vi "module-07-sample-7-1-ALT2.vi"() -> ()   [LabVIEW 2019]
uses:
  CubeGrabeState_ENUM.ctl
  <vilib>/Rock Robotics/WPI/ThirdParty/JAS_Junk/TrajLib/Trajectory_Library.lvlib
  samples-common-library/Ctrl_Training_Library_Protected/CtrlTrainingLibary_Protected.lvlib
panel:
  in  "Tab Control":T1(tab)
  in  "Driver Gather Cube":bool
  in  "Driver Cancel Button":bool
  out "Request GO":bool
  out "Digital State Chart":cluster{dbl, dbl, dbl, dbl, dbl, dbl}(graph)
  out "Ready":bool
  out "Arm Extend Cmd":bool
  out "Hand Close Cmd":bool
  out "State":i32
  out "Done Time":dbl format="%20.3f"
  out "Cur Time":dbl format="%20.3f"
  out "State Text":T2
  # "Training Sample 7.1  ALT 2\nState Machine"
  # "F1"
  # "F2"
  # "NOTE: Outer loop not shown for simplicity"
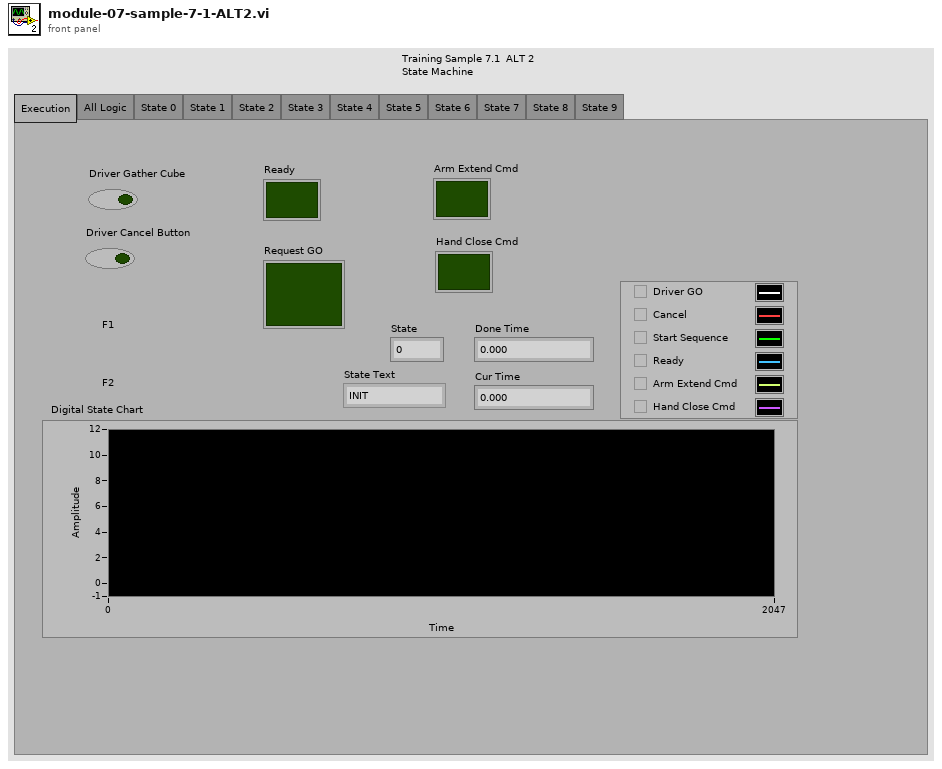
[diagram p1: front panel]
types:
  T1 = enum32{"Execution", "All Logic", "State 0", "State 1", "State 2", "State 3", "State 4", "State 5", "State 6", "State 7", "State 8", "State 9"}
  T2 = typedef "CubeGrabeState_ENUM.ctl" = enum16{"INIT", "ArmExtend", "ArmExtendWait", "HandClose", "HandCloseWait", "ArmRetract", "ArmRetractWait", "HandOpen", "HandOpenWait", "Ready"}
  T3 = typedef "Trajectory_Library.lvlib/TIMER.ctl" = cluster{"StartTime":dbl, "Accumulated TIme":dbl, "Running":bool, "semaphore":T4}
  T4 = typedef "Semaphore RefNum" = refnum<k1>
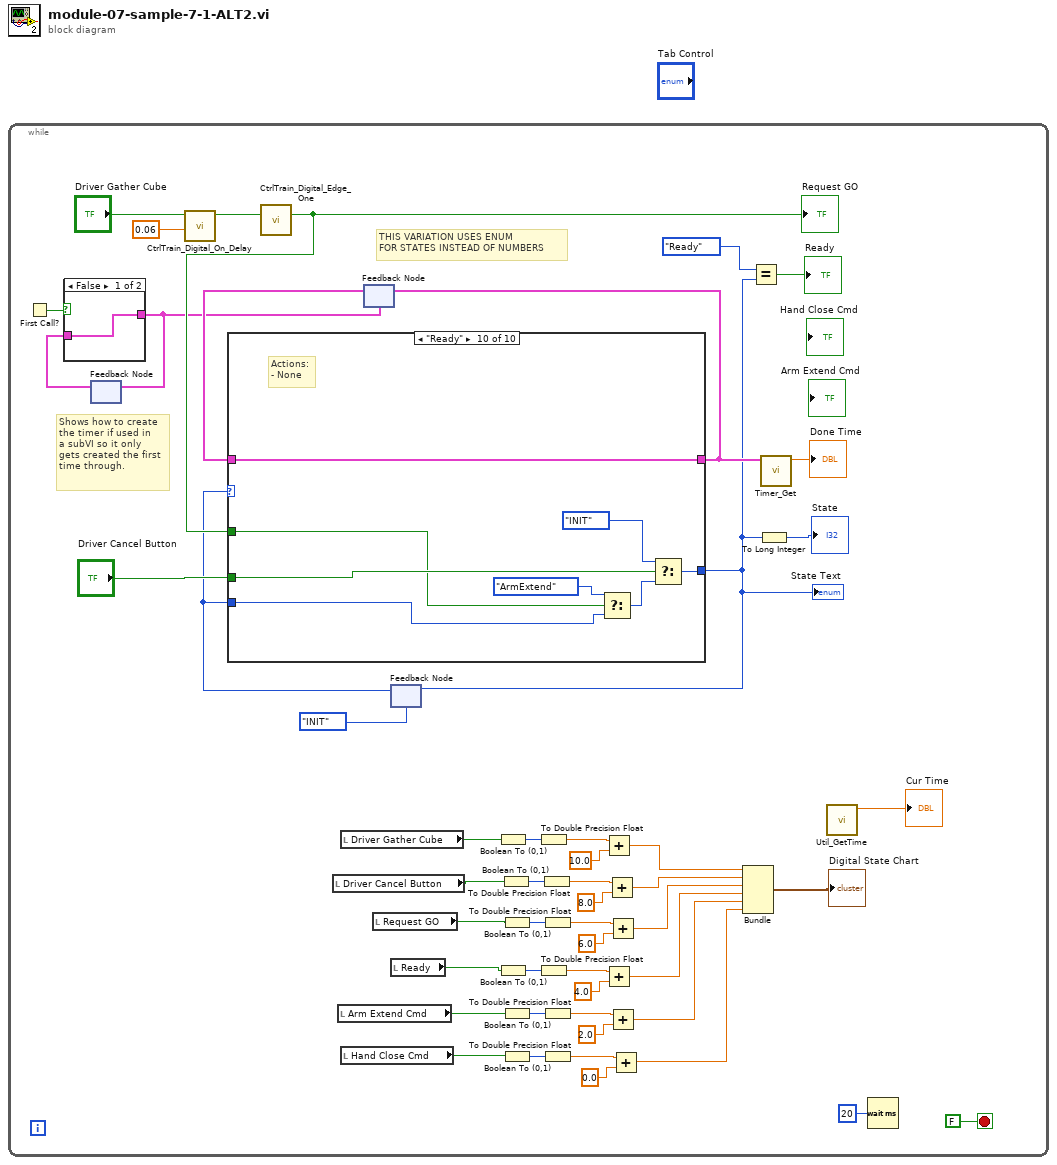
[diagram p0: block diagram]
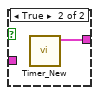
[diagram p2: hidden frame]
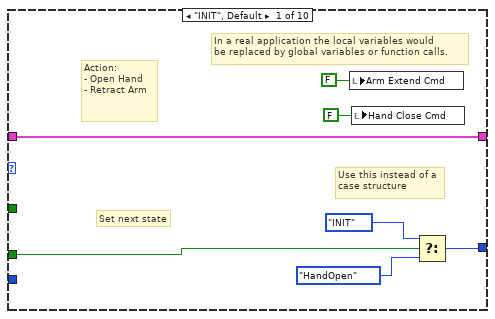
[diagram p3: hidden frame]
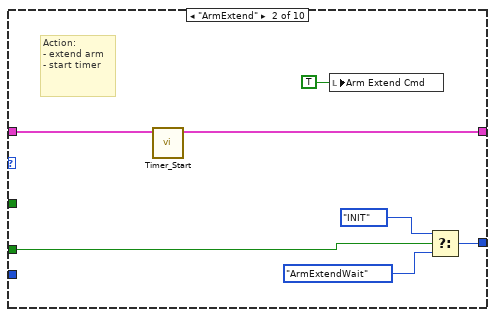
[diagram p4: hidden frame]
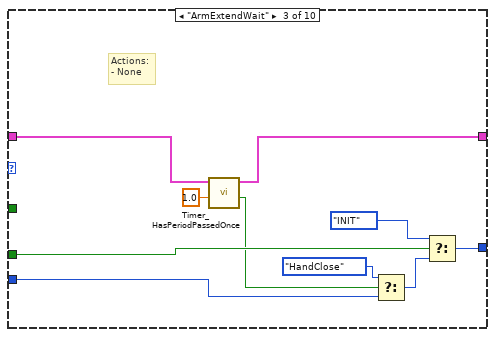
[diagram p5: hidden frame]
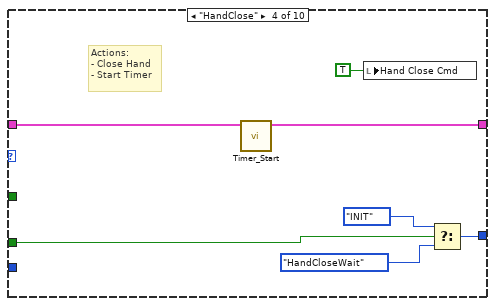
[diagram p6: hidden frame]
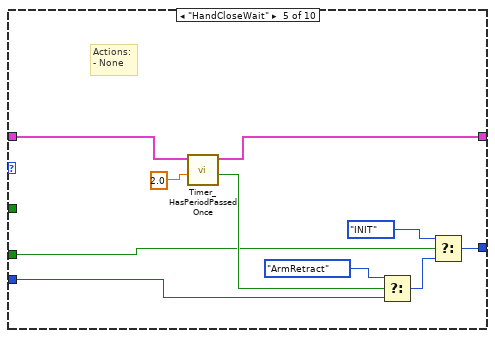
[diagram p7: hidden frame]
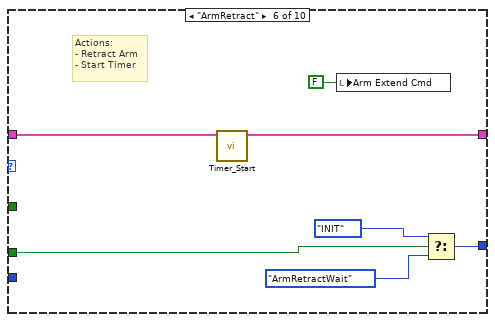
[diagram p8: hidden frame]
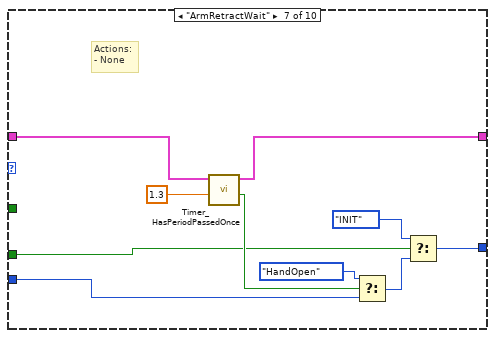
[diagram p9: hidden frame]
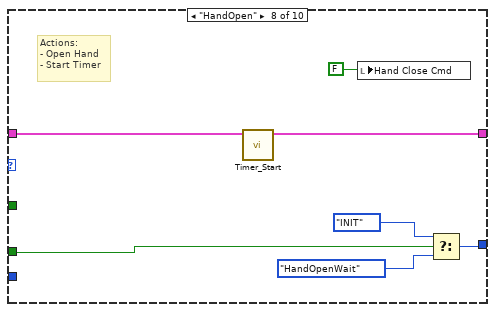
[diagram p10: hidden frame]
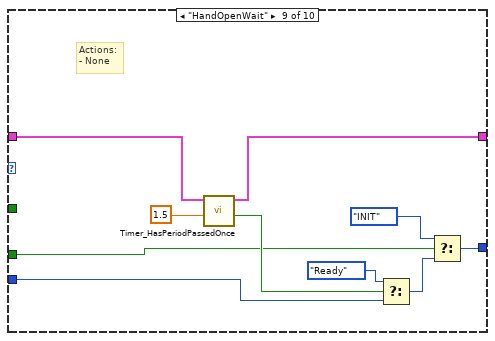
[diagram p11: hidden frame]
diagram:
  n1 = while {
    stop <- FALSE stop-if-true
    # "THIS VARIATION USES ENUM\nFOR STATES INSTEAD OF NUMBERS"
    # "Shows how to create\nthe timer if used in\na subVI so it only\ngets created the first\ntime through."
    n2 = First Call?() -> (First Call?: T/F=w9:bool)
    n3 = feedback #1() -> (w7:T3)  [unwired: 1 in]
    n4 = case shown="False" w9 {
      tunnel: [w52 w53] -> w8
      tunnel: w7 -> [w52 _]
      frame False {
      }
      frame True {
        n5 = call <vilib>:"Timer_New.vi"() -> ("TIMER"=w53:T3)  [unwired: 11 in]
      }
    }
    n6 = feedback-in #1(w8) -> ()
    n7 = call "CtrlTrain_Digital_On_Delay.vi"("Delay"=0.06, "Input"="Driver Gather Cube") -> ("Output"=w17:bool)  [unwired: 8 in, 1 out]
    n8 = call "CtrlTrain_Digital_Edge_One.vi"("Input"=w17) -> ("Output"=w13:bool)  [unwired: 14 in]
    "Request GO" <- w13
    n9 = local read "Driver Cancel Button"() -> (w6:bool)
    n10 = local read "Arm Extend Cmd"() -> (w22:bool)
    n11 = local read "Driver Gather Cube"() -> (w24:bool)
    n12 = local read "Hand Close Cmd"() -> (w23:bool)
    n13 = feedback #2(w8) -> (w19:T3)
    n14 = local read "Request GO"() -> (w21:bool)
    n15 = feedback #3(CubeGrabeState_ENUM."INIT") -> (w5:T2)
    n16 = case shown="\"Ready\"" w5 {
      tunnel: [w58 w64 w75 w82 w92 w100 w110 w116 w127 w136] -> w11
      tunnel: w19 -> [w58 w65 w77 w83 w93 w99 w111 w117 w128 w136]
      tunnel: w5 -> [_ _ w70 _ w86 _ w103 _ w122 w131]
      tunnel: "Driver Cancel Button" -> [w57 w66 w74 w81 w89 w98 w107 w115 w124 w135]
      tunnel: w13 -> [_ _ _ _ _ _ _ _ _ w134]
      tunnel: [w54 w61 w68 w78 w85 w95 w102 w112 w119 w129] -> w1
      frame "INIT", Default {
        # "In a real application the local variables would\nbe replaced by global variables or function calls."
        # "Use this instead of a\ncase structure"
        # "Set next state"
        # "Action:\n- Open Hand \n- Retract Arm"
        n17 = local write "Arm Extend Cmd"(FALSE ("Arm Extend Cmd")) -> ()
        n18 = local write "Hand Close Cmd"(FALSE ("Hand Close Cmd")) -> ()
        n19 = Select(t=CubeGrabeState_ENUM."INIT", s=w57, f=CubeGrabeState_ENUM."HandOpen") -> (s? t:f=w54:T2)
      }
      frame "ArmExtend" {
        # "Action:\n- extend arm \n- start timer"
        n20 = call <vilib>:"Timer_Start.vi"("in Timer"=w65) -> ("out Timer"=w64:T3)  [unwired: 10 in]
        n21 = local write "Arm Extend Cmd"(TRUE ("Arm Extend Cmd")) -> ()
        n22 = Select(t=CubeGrabeState_ENUM."INIT", s=w66, f=CubeGrabeState_ENUM."ArmExtendWait") -> (s? t:f=w61:T2)
      }
      frame "ArmExtendWait" {
        # "Actions:\n- None"
        n23 = call <vilib>:"Timer_HasPeriodPassedOnce.vi"("Period"=1.0, "in Timer"=w77) -> ("Expired"=w73:bool, "out Timer"=w75:T3)  [unwired: 7 in, 1 out]
        n24 = Select(t=CubeGrabeState_ENUM."HandClose", s=w73, f=w70) -> (s? t:f=w69:T2)
        n25 = Select(t=CubeGrabeState_ENUM."INIT", s=w74, f=w69) -> (s? t:f=w68:T2)
      }
      frame "HandClose" {
        # "Actions:\n- Close Hand\n- Start Timer"
        n26 = call <vilib>:"Timer_Start.vi"("in Timer"=w83) -> ("out Timer"=w82:T3)  [unwired: 10 in]
        n27 = local write "Hand Close Cmd"(TRUE ("Hand Close Cmd")) -> ()
        n28 = Select(t=CubeGrabeState_ENUM."INIT", s=w81, f=CubeGrabeState_ENUM."HandCloseWait") -> (s? t:f=w78:T2)
      }
      frame "HandCloseWait" {
        # "Actions:\n- None"
        n29 = call <vilib>:"Timer_HasPeriodPassedOnce.vi"("Period"=2.0 ("Elapsed"), "in Timer"=w93) -> ("Expired"=w90:bool, "out Timer"=w92:T3)  [unwired: 7 in, 1 out]
        n30 = Select(t=CubeGrabeState_ENUM."ArmRetract", s=w90, f=w86) -> (s? t:f=w91:T2)
        n31 = Select(t=CubeGrabeState_ENUM."INIT", s=w89, f=w91) -> (s? t:f=w85:T2)
      }
      frame "ArmRetract" {
        # "Actions:\n- Retract Arm\n- Start Timer"
        n32 = call <vilib>:"Timer_Start.vi"("in Timer"=w99) -> ("out Timer"=w100:T3)  [unwired: 10 in]
        n33 = local write "Arm Extend Cmd"(FALSE ("Arm Extend Cmd")) -> ()
        n34 = Select(t=CubeGrabeState_ENUM."INIT", s=w98, f=CubeGrabeState_ENUM."ArmRetractWait") -> (s? t:f=w95:T2)
      }
      frame "ArmRetractWait" {
        # "Actions:\n- None"
        n35 = call <vilib>:"Timer_HasPeriodPassedOnce.vi"("Period"=1.3 ("Elapsed"), "in Timer"=w111) -> ("Expired"=w108:bool, "out Timer"=w110:T3)  [unwired: 7 in, 1 out]
        n36 = Select(t=CubeGrabeState_ENUM."HandOpen", s=w108, f=w103) -> (s? t:f=w104:T2)
        n37 = Select(t=CubeGrabeState_ENUM."INIT", s=w107, f=w104) -> (s? t:f=w102:T2)
      }
      frame "HandOpen" {
        # "Actions:\n- Open Hand\n- Start Timer"
        n38 = call <vilib>:"Timer_Start.vi"("in Timer"=w117) -> ("out Timer"=w116:T3)  [unwired: 10 in]
        n39 = local write "Hand Close Cmd"(FALSE ("Hand Close Cmd")) -> ()
        n40 = Select(t=CubeGrabeState_ENUM."INIT", s=w115, f=CubeGrabeState_ENUM."HandOpenWait") -> (s? t:f=w112:T2)
      }
      frame "HandOpenWait" {
        # "Actions:\n- None"
        n41 = call <vilib>:"Timer_HasPeriodPassedOnce.vi"("Period"=1.5 ("Elapsed"), "in Timer"=w128) -> ("Expired"=w125:bool, "out Timer"=w127:T3)  [unwired: 7 in, 1 out]
        n42 = Select(t=CubeGrabeState_ENUM."Ready", s=w125, f=w122) -> (s? t:f=w121:T2)
        n43 = Select(t=CubeGrabeState_ENUM."INIT", s=w124, f=w121) -> (s? t:f=w119:T2)
      }
      frame "Ready" {
        # "Actions:\n- None"
        n44 = Select(t=CubeGrabeState_ENUM."ArmExtend", s=w134, f=w131) -> (s? t:f=w130:T2)
        n45 = Select(t=CubeGrabeState_ENUM."INIT", s=w135, f=w130) -> (s? t:f=w129:T2)
      }
    }
    "State Text" <- w1
    n46 = feedback-in #2(w11) -> ()
    n47 = feedback-in #3(w1) -> ()
    n48 = local read "Ready"() -> (w20:bool)
    n49 = Boolean To (0,1)(Boolean=w24) -> (0, 1=w49:i16)
    n50 = Boolean To (0,1)(Boolean=w20) -> (0, 1=w47:i16)
    n51 = Boolean To (0,1)(Boolean=w6) -> (0, 1=w44:i16)
    n52 = Boolean To (0,1)(Boolean=w21) -> (0, 1=w41:i16)
    n53 = Boolean To (0,1)(Boolean=w22) -> (0, 1=w38:i16)
    n54 = Boolean To (0,1)(Boolean=w23) -> (0, 1=w35:i16)
    n55 = To Double Precision Float(number=w49) -> (double precision float=w26:dbl)
    n56 = To Double Precision Float(number=w47) -> (double precision float=w46:dbl)
    n57 = To Double Precision Float(number=w44) -> (double precision float=w43:dbl)
    n58 = To Double Precision Float(number=w41) -> (double precision float=w40:dbl)
    n59 = To Double Precision Float(number=w38) -> (double precision float=w37:dbl)
    n60 = To Double Precision Float(number=w35) -> (double precision float=w34:dbl)
    n61 = Add(x=w26, y=10.0) -> (x+y=w25:dbl)
    n62 = Add(x=w46, y=4.0) -> (x+y=w29:dbl)
    n63 = Add(x=w43, y=8.0) -> (x+y=w31:dbl)
    n64 = Add(x=w40, y=6.0) -> (x+y=w30:dbl)
    n65 = Add(x=w37, y=2.0) -> (x+y=w33:dbl)
    n66 = Add(x=w34, y=0.0) -> (x+y=w32:dbl)
    n67 = Bundle(w25, w31, w30, w29, w33, w32) -> (→"Digital State Chart":cluster{dbl, dbl, dbl, dbl, dbl, dbl})  [unwired: 1 in]
    n68 = Equal?(x=CubeGrabeState_ENUM."Ready", y=w1) -> (x = y?=→"Ready":bool)
    n69 = To Long Integer(number=w1) -> (32bit integer=→"State":i32)
    n70 = call <vilib>:"Timer_Get.vi"("TIMER"=w11) -> ("CurrentTImer"=→"Done Time":dbl)  [unwired: 10 in]
    n71 = call <vilib>:"Util_GetTime.vi"() -> ("FPGA_Time_Seconds"=→"Cur Time":dbl)  [unwired: 10 in, 1 out]
    n72 = Wait (ms)(milliseconds to wait=u32 20) -> ()  [unwired: 1 out]
  }
